vi "Initialize.vi"(11 "Serial Number":i32) -> (0 "error out":errorcluster, 3 "reference out":refnum<k7>)   [LabVIEW 2020, in "Shutter.lvlib"]
uses:
  Shutter.lvlib
panel:
  in  "MG17Motor":refnum<k7>(container)
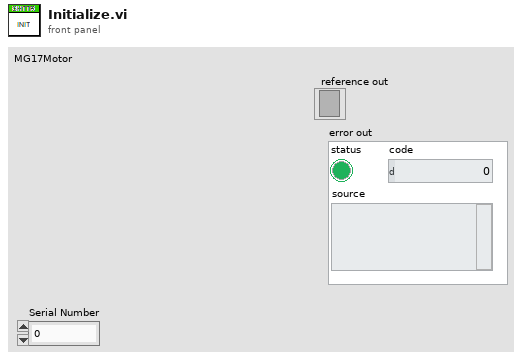
[diagram p1: front panel]
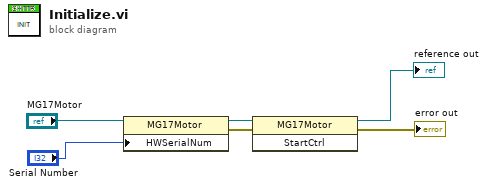
[diagram p0: block diagram]
diagram:
  n1 = property class="MG17Motor"(reference="MG17Motor", "HWSerialNum"="Serial Number") -> (reference out=w5:refnum<k7>, error out=w6:errorcluster)  [unwired: 1 in]
  n2 = invoke class="MG17Motor" method="StartCtrl"(reference=w5, error in=w6) -> (reference out=→"reference out":refnum<k7>, error out=→"error out":errorcluster)  [unwired: 1 in, 1 out]
